vi "Soft Front Panel.vi"(8 "error in (no error)":errorcluster, 10 "SubPanel Ref":i32, 11 "Instrument in":refnum<class "Instrument.lvclass">) -> (0 "error out":errorcluster, 3 "Instrument out":refnum<class "Instrument.lvclass">)   [LabVIEW 2015, in "Instrument.lvlib" / "Instrument.lvclass"]
uses:
  Instrument.lvclass
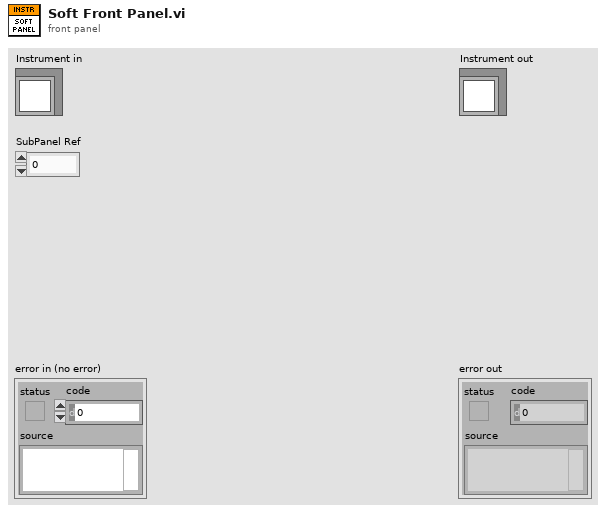
[diagram p1: front panel]
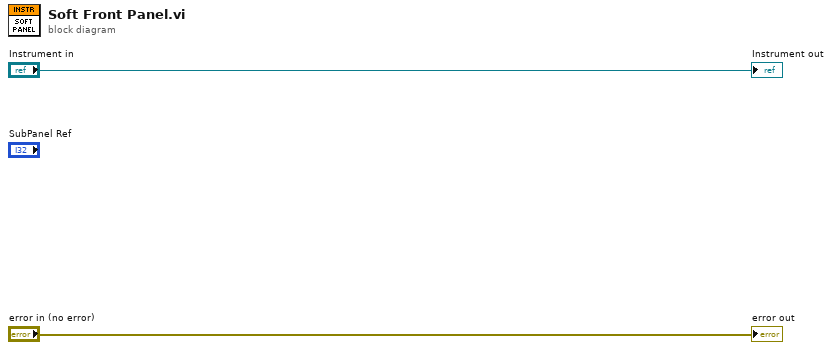
[diagram p0: block diagram]
diagram:
  "error out" <- "error in (no error)"
  "Instrument out" <- "Instrument in"
